vi "Wavegen turn on.vi"(8 "error in (no error)":errorcluster, 9 "Output Enabled (TRUE)":bool=TRUE, 11 "IVI Refnum in":refnum<k15>) -> (0 "error out":errorcluster, 2 "log string out":string, 3 "IVI Refnum out":refnum<k15>)   [LabVIEW 2021]
uses:
  <instrlib>/Keysight InfiniiVision/Keysight InfiniiVision.lvlib
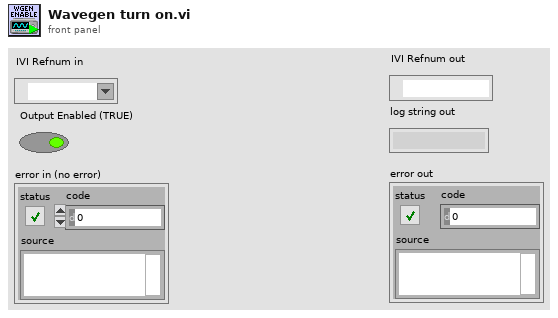
[diagram p1: front panel]
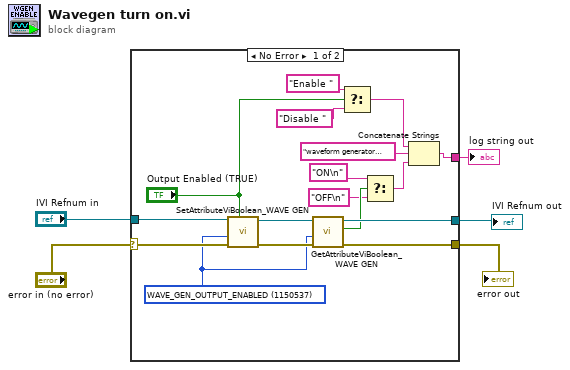
[diagram p0: block diagram]
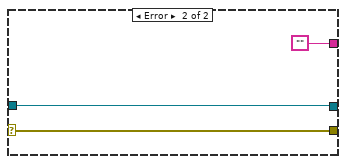
[diagram p2: hidden frame]
diagram:
  n1 = case shown="No Error" "error in (no error)" {
    selector: "error in (no error)" -> [w21 w24]
    tunnel: "IVI Refnum in" -> [w22 w25]
    tunnel: [w17 w24] -> w4
    tunnel: [w18 w25] -> w3
    tunnel: [w10 ""] -> w1
    frame No Error {
      w16 = u32 1150537 items=["ARBITRARY_INTERPOLATION"=1150411, "MODULATION_ENABLED"=1150554, "TRACKING_AMPLITUDE"=1150527, "TRACKING_ENABLED"=1150526, "TRACKING_FREQUENCY"=1150528, "WAVE_GEN_ARBITRARY_INTERPOLATION"=1150543, "WAVE_GEN_OUTPUT_ENABLED"=1150537, "WAVE_GEN_OUTPUT_INVERTED"=1150545] ("AttributeID")
      n2 = call <instrlib>:"SetAttributeViBoolean_WAVE GEN.vi"("AttributeValue (Off)"="Output Enabled (TRUE)", "error in (no error)"=w21, "AttributeID"=w16, "instrument handle"=w22) -> ("error out"=w19:errorcluster, "instrument handle out"=w20:refnum<k15>)  [unwired: 6 in]
      n3 = call <instrlib>:"GetAttributeViBoolean_WAVE GEN.vi"("error in (no error)"=w19, "AttributeID"=w16, "instrument handle"=w20) -> ("error out"=w17:errorcluster, "AttributeValue"=w15:bool, "instrument handle out"=w18:refnum<k15>)  [unwired: 6 in]
      n4 = Select(t="Enable ", s="Output Enabled (TRUE)", f="Disable ") -> (s? t:f=w7:string)
      n5 = Select(t="ON\n", s=w15, f="OFF\n") -> (s? t:f=w12:string)
      n6 = Concatenate Strings(w7, "waveform generator output\nOutput: " ("string"), w12) -> (w10:string)
    }
    frame Error {
    }
  }
  "error out" <- w4
  "IVI Refnum out" <- w3
  "log string out" <- w1
